vi "Get_Initial_Tracks_and_Separate_on_Duration-4.vi"(3 "error IN":errorcluster, 4 "dR max":dbl, 5 "dR min":dbl, 6 "[IN] Potential\nMoving Dots (X,Y)":dbl[][](array[numeric])) -> (0 "error OUT":errorcluster, 1 "Displacements =1 Frame":dbl[][](array[numeric]), 2 "Displacements >1 Frame":dbl[][](array[numeric]))   [LabVIEW 2013]
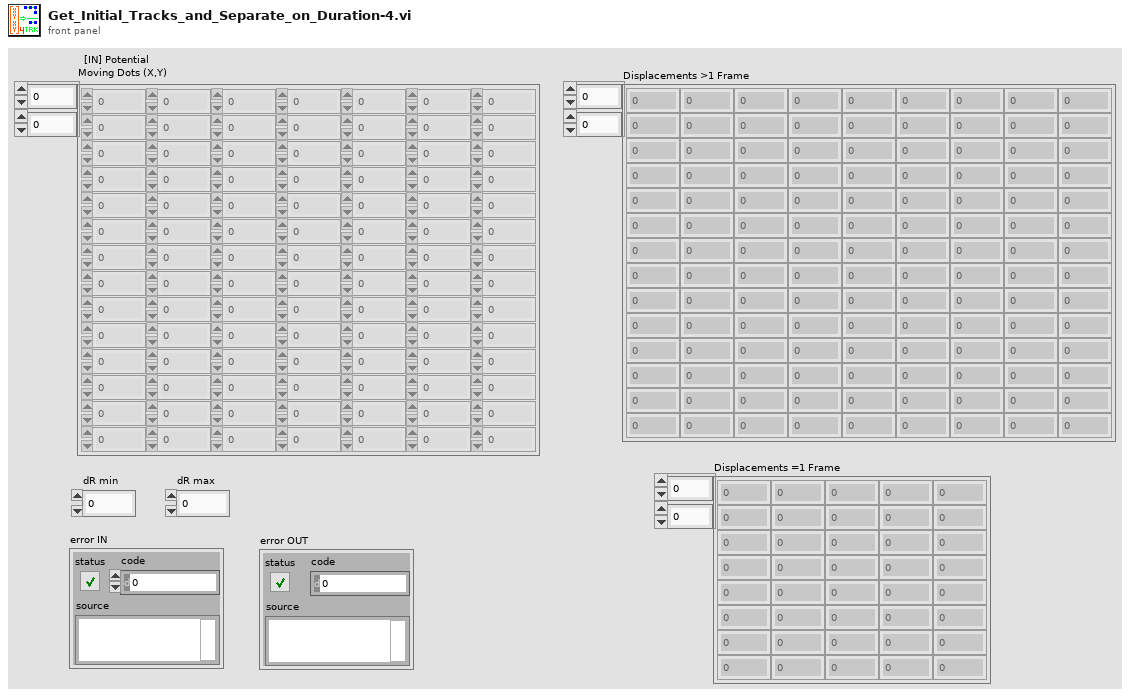
[diagram p1: front panel]
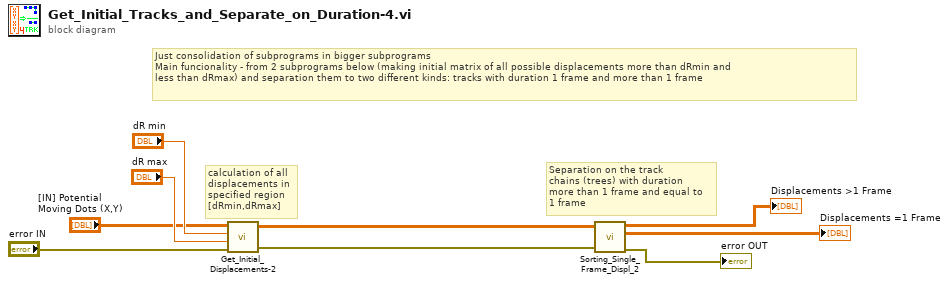
[diagram p0: block diagram]
diagram:
  # "Just consolidation of subprograms in bigger subprograms\nMain funcionality - from 2 subprograms below (making initial matrix of all possible displacements more than dRmin and\nless than dRmax) and separation them to two different kinds: tracks with duration 1 frame and more than 1 frame"
  # "Separation on the track\nchains (trees) with duration\nmore than 1 frame and equal to \n1 frame"
  # "calculation of all \ndisplacements in\nspecified region \n[dRmin,dRmax]"
  n1 = call "Get_Initial_Displacements-2.vi"("error IN"="error IN", "dR max"="dR max", "dR min"="dR min", "[IN] (X,Y)"="[IN] Potential\nMoving Dots (X,Y)") -> ("error OUT"=w1:errorcluster, "[OUT] Raw Displacements"=w2:dbl[][])  [unwired: 1 in]
  n2 = call "Sorting_Single_Frame_Displ_2.vi"("(X,Y,dX,dY) IN"=w2, "error IN"=w1) -> ("Displ >1 Frame"=→"Displacements >1 Frame":dbl[][], "Displ =1 Frame"=→"Displacements =1 Frame":dbl[][], "error OUT"=→"error OUT":errorcluster)  [unwired: 2 in]
